vi "Warn when below specified thresgold.vi"(0 "base path":path, 5 "Warning Trigger set (in)":bool, 7 "Critical Trigger set (in)":bool, 9 "Warning threshold %":i32, 11 "Critical threshold %":i32) -> (1 "path out":path, 2 "Critical Limit (GB)":dbl, 3 "size (GB)":dbl, 4 "Warning Limit (GB)":dbl, 6 "Warning Trigger set (out)":bool, 8 "Critical Trigger set (out)":bool, 10 "free (GB)":dbl, 12 "Below critical threshold":bool, 14 "Below warning threshold":bool, 15 "error out":errorcluster)   [LabVIEW 2020]
panel:
  in  "Demo":dbl(knob)=796137.0075332791
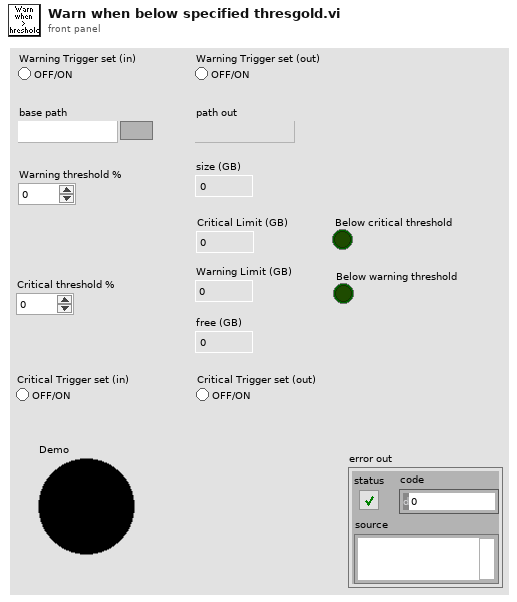
[diagram p1: front panel]
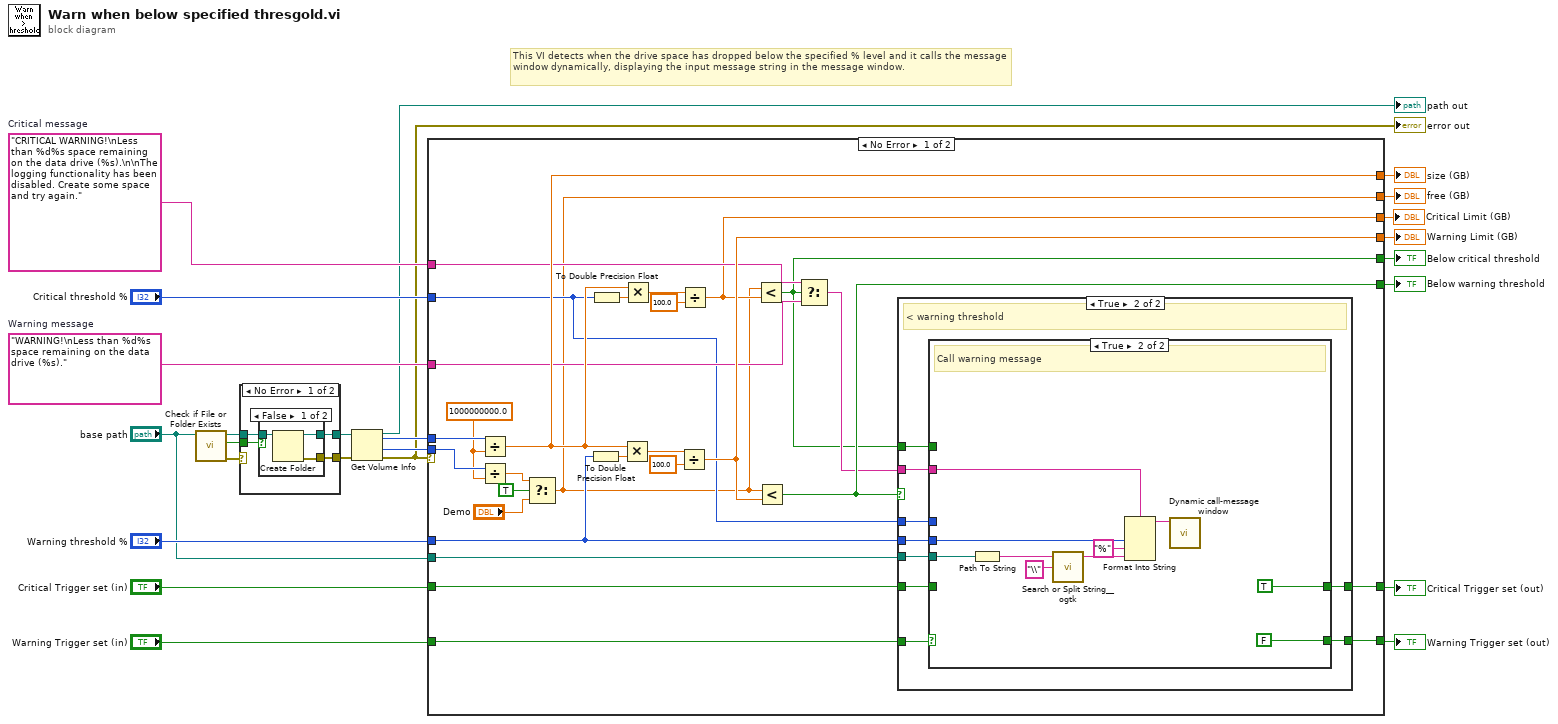
[diagram p0: block diagram]
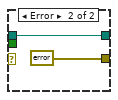
[diagram p3: hidden frame]
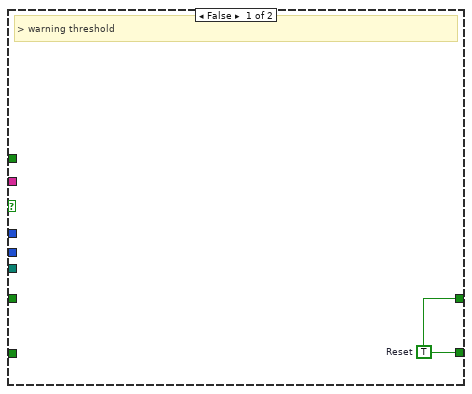
[diagram p4: hidden frame]
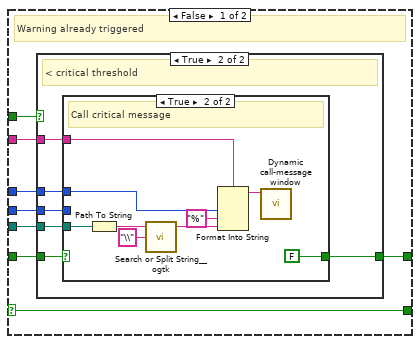
[diagram p5: hidden frame]
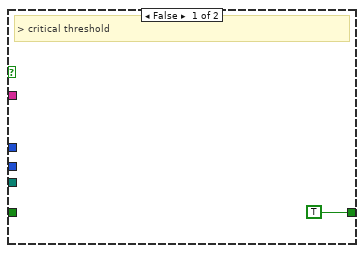
[diagram p6: hidden frame]
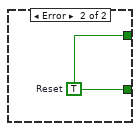
[diagram p8: hidden frame]
diagram:
  w9 = "CRITICAL WARNING!\nLess than %d%s space remaining on the data drive (%s).\n\nThe logging functionality has been disabled. Create some space and try again."  # Critical message
  w13 = "WARNING!\nLess than %d%s space remaining on the data drive (%s)."  # Warning message
  # "This VI detects when the drive space has dropped below the specified % level and it calls the message window dynamically, displaying the input message string in the message window."
  n1 = call <vilib>:"Check if File or Folder Exists.vi"("path"="base path") -> ("error out"=w3:errorcluster, "file or folder exists?"=w1:bool, "dup path"=w4:path)  [unwired: 8 in]
  n2 = case shown="No Error" w3 {
    tunnel: [w28 w34] -> w6
    tunnel: w4 -> [w27 w34]
    tunnel: [w26 errorcluster {"status"=FALSE, "code"=0, "source"=""} ("error out")] -> w2
    tunnel: w1 -> [w25 _]
    frame No Error {
      n3 = case shown="False" w25 {
        tunnel: [w31 w32] -> w28
        tunnel: w27 -> [w30 w32]
        tunnel: [w29 _] -> w26
        frame False {
          n4 = Create Folder(path (use dialog)=w30) -> (created path=w31:path, error out=w29:errorcluster)  [unwired: 2 in, 1 out]
        }
        frame True {
        }
      }
    }
    frame Error {
    }
  }
  n5 = Get Volume Info(8:w2, 11:w6) -> (0:w8:errorcluster, 1:w21:i64, 2:w20:i64, 3:→"path out":path)  [unwired: 2 out]
  "error out" <- w8
  n6 = case shown="No Error" w8 {
    tunnel: w20 -> [w62 _]
    tunnel: w21 -> [w61 _]
    tunnel: "Warning threshold %" -> [w56 _]
    tunnel: "base path" -> [w55 _]
    tunnel: [w54 w108] -> w23
    tunnel: "Warning Trigger set (in)" -> [w53 _]
    tunnel: [w47 _] -> w19
    tunnel: [w37 _] -> w18
    tunnel: [w52 _] -> w17
    tunnel: [w51 _] -> w16
    tunnel: "Critical threshold %" -> [w39 _]
    tunnel: w13 -> [w46 _]
    tunnel: w9 -> [w45 _]
    tunnel: [w43 _] -> w14
    tunnel: "Critical Trigger set (in)" -> [w42 _]
    tunnel: [w41 w108] -> w11
    tunnel: [w40 _] -> w10
    frame No Error {
      w60 = 1000000000.0 ("y")
      n7 = Divide(x=w62, y=w60) -> (x/y=w47:dbl)
      n8 = Divide(x=w61, y=w60) -> (x/y=w38:dbl)
      n9 = Select(t=w38, s=TRUE, f="Demo") -> (s? t:f=w37:dbl)
      n10 = To Double Precision Float(number=w56) -> (double precision float=w57:dbl)
      n11 = To Double Precision Float(number=w39) -> (double precision float=w50:dbl)
      n12 = Multiply(x=w47, y=w57) -> (x*y=w59:dbl)
      n13 = Multiply(x=w47, y=w50) -> (x*y=w48:dbl)
      n14 = Divide(x=w59, y=100.0) -> (x/y=w52:dbl)
      n15 = Divide(x=w48, y=100.0) -> (x/y=w40:dbl)
      n16 = Less?(x=w37, y=w40) -> (x < y?=w43:bool)
      n17 = Less?(x=w37, y=w52) -> (x < y?=w51:bool)
      n18 = Select(t=w45, s=w43, f=w46) -> (s? t:f=w44:string)
      n19 = case shown="True" w51 {
        tunnel: w56 -> [_ w72]
        tunnel: w55 -> [_ w71]
        tunnel: [w63 w70] -> w54
        tunnel: w53 -> [_ w69]
        tunnel: w44 -> [_ w68]
        tunnel: w43 -> [_ w67]
        tunnel: w42 -> [_ w66]
        tunnel: [w63 w65] -> w41
        tunnel: w39 -> [_ w64]
        frame False {
          w63 = TRUE  # Reset
          # "> warning threshold"
        }
        frame True {
          # "< warning threshold"
          n20 = case shown="True" w69 {
            selector: w69 -> [w75 _]
            tunnel: w72 -> [w78 w107]
            tunnel: w71 -> [w80 w104]
            tunnel: [w75 FALSE] -> w70
            tunnel: w68 -> [w79 w99]
            tunnel: w67 -> [w77 _]
            tunnel: w66 -> [w76 _]
            tunnel: [w74 TRUE] -> w65
            tunnel: w64 -> [w73 _]
            frame False {
              # "Warning already triggered"
              n21 = case shown="True" w77 {
                tunnel: w78 -> [_ w87]
                tunnel: w80 -> [_ w86]
                tunnel: w79 -> [_ w85]
                tunnel: w76 -> [_ w84]
                tunnel: [TRUE w83] -> w74
                tunnel: w73 -> [_ w82]
                frame False {
                  # "> critical threshold"
                }
                frame True {
                  # "< critical threshold"
                  n22 = case shown="True" w84 {
                    selector: w84 -> [w88 _]
                    tunnel: w87 -> [_ _]
                    tunnel: w86 -> [_ w95]
                    tunnel: w85 -> [_ w91]
                    tunnel: [w88 FALSE] -> w83
                    tunnel: w82 -> [_ w89]
                    frame False {
                      # "Critical already triggered"
                    }
                    frame True {
                      # "Call critical message"
                      n23 = Path To String(path=w95) -> (string=w97:string)
                      n24 = call <userlib>:"Search or Split String__ogtk.vi"("search string/char (-)"="\\", "string"=w97) -> ("substring before match"=w93:string)  [unwired: 1 in, 2 out]
                      n25 = Format Into String(format string=w91, w89, "%" ("input 2"), w93) -> (resulting string=w94:string)  [unwired: 2 in, 1 out]
                      n26 = call "Dynamic call-message window.vi"("Message"=w94) -> ()  [unwired: 10 in, 1 out]
                    }
                  }
                }
              }
            }
            frame True {
              # "Call warning message"
              n27 = Path To String(path=w104) -> (string=w106:string)
              n28 = call <userlib>:"Search or Split String__ogtk.vi"("search string/char (-)"="\\", "string"=w106) -> ("substring before match"=w102:string)  [unwired: 1 in, 2 out]
              n29 = Format Into String(format string=w99, w107, "%" ("input 2"), w102) -> (resulting string=w103:string)  [unwired: 2 in, 1 out]
              n30 = call "Dynamic call-message window.vi"("Message"=w103) -> ()  [unwired: 10 in, 1 out]
            }
          }
        }
      }
    }
    frame Error {
      w108 = TRUE  # Reset
    }
  }
  "Warning Trigger set (out)" <- w23
  "size (GB)" <- w19
  "free (GB)" <- w18
  "Warning Limit (GB)" <- w17
  "Below warning threshold" <- w16
  "Below critical threshold" <- w14
  "Critical Trigger set (out)" <- w11
  "Critical Limit (GB)" <- w10
